vi "openTiffImage.vi"(8 "error in (no error)":errorcluster, 11 "NewVal":path) -> (0 "error out":errorcluster, 3 "returned pointer":i64)   [LabVIEW 2013]
uses:
  imagereconstruction/x64/Debug/labviewdll.dll
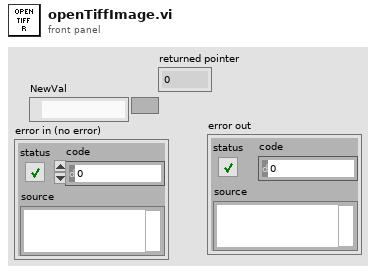
[diagram p1: front panel]
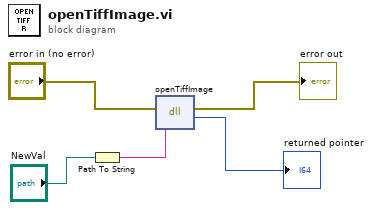
[diagram p0: block diagram]
diagram:
  n1 = Path To String(path="NewVal") -> (string=w5:string)
  n2 = dll-call lib="D:/work/uni/FYP/reconrepo/imagereconstruction/x64/Debug/labviewdll.dll" fn="openTiffImage"(error in="error in (no error)", "path"=w5) -> (error out=→"error out":errorcluster, "return type"=→"returned pointer":i64)  [unwired: 3 in, 1 out]
